vi "Core-GetTicks.vi"(8 "error in (no error)":errorcluster, 11 "Engine in":refnum<class "Engine.lvclass">) -> (0 "error out":errorcluster, 3 "Engine out":refnum<class "Engine.lvclass">)   [LabVIEW 2024, in "GLF.lvlib" / "Engine.lvclass"]
uses:
  Engine.lvclass
  Engine.lvclass/Engine.ctl
  <vilib>/Saukko/LV SDL3/Sources/SDL3/Timer/Timer.lvlib
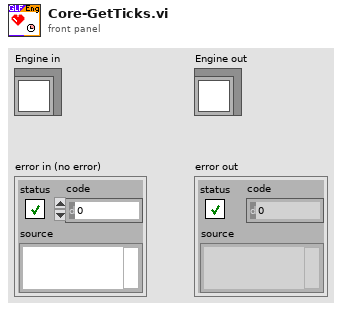
[diagram p1: front panel]
types:
  T1 = typedef "GLF.lvlib/Engine.lvclass/DVR--cluster.ctl" = cluster{"CMD Queue":T2, "Config":T3, "Ctxt":T5, "Metrics":T6, "GLF Instances":set{refnum<class "IAmGLF.lvclass">}, "Window Instances":map{i64, refnum<class "Window.lvclass">}}
  T2 = typedef "GLF.lvlib/Engine.lvclass/Command--queue.ctl" = refnum<queue>
  T3 = typedef "GLF.lvlib/Engine.lvclass/Config--cluster.ctl" = cluster{"Quit On Last Window Closed":bool, "VSync":T4, "FPS Target":dbl}
  T4 = typedef "GLF.lvlib/Engine.lvclass/VSync--enum.ctl" = enum16{"Disabled", "Enabled", "Adaptative"}
  T5 = typedef "GLF.lvlib/Engine.lvclass/Context--cluster.ctl" = cluster{"Ticks Begin":u64, "VSync Enabled":bool}
  T6 = typedef "GLF.lvlib/Engine.lvclass/Metrics--cluster.ctl" = cluster{"Uptime [ms]":u64, "Loop Time [ms]":u64}
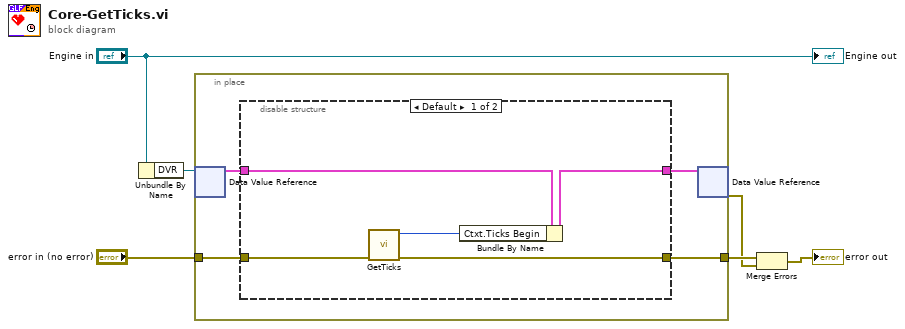
[diagram p0: block diagram]
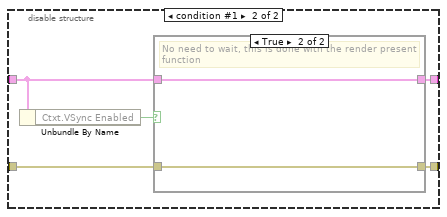
[diagram p2: hidden frame]
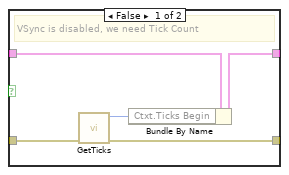
[diagram p3: hidden frame]
diagram:
  n1 = Unbundle By Name("Engine in") -> ("DVR"=w3:refnum<data-value>)
  n2 = in-place {
    in-place-border: "error in (no error)" -> [w10]
    in-place-border: [w9] -> w5
    n3 = in-place-dvr #1(w3) -> (w8:T1)  [unwired: 1 out]
    n4 = disable-structure shown="Default" {
      disable-tunnel: w10 -> [w15 w20]
      disable-tunnel: w8 -> [w12 w17]
      disable-tunnel: [w11 w19] -> w7
      disable-tunnel: [w13 w18] -> w9
      frame condition #0 (active) {
        n5 = call <vilib>:"GetTicks.vi"("No Error"=w15) -> ("error out"=w13:errorcluster, "Ticks [ms]"=w14:u64)  [unwired: 9 in]
        n6 = Bundle By Name(cluster=w12, "Ctxt.Ticks Begin"=w14) -> (w11:T1)
      }
      frame condition #1 {
        n7 = Unbundle By Name(w17) -> ("Ctxt.VSync Enabled"=w16:bool)
        n8 = case shown="True" w16 {
          tunnel: w20 -> [w25 w26]
          tunnel: w17 -> [w24 w27]
          tunnel: [w23 w27] -> w19
          tunnel: [w21 w26] -> w18
          frame False {
            # "VSync is disabled, we need Tick Count"
            n9 = call <vilib>:"GetTicks.vi"("No Error"=w25) -> ("error out"=w21:errorcluster, "Ticks [ms]"=w22:u64)  [unwired: 9 in]
            n10 = Bundle By Name(cluster=w24, "Ctxt.Ticks Begin"=w22) -> (w23:T1)
          }
          frame True {
            # "No need to wait, this is done with the render present function"
          }
        }
      }
    }
    n11 = in-place-dvr #1(w7) -> (w1:errorcluster)  [unwired: 1 out]
  }
  n12 = Merge Errors(w5, w1) -> (→"error out":errorcluster)
  "Engine out" <- "Engine in"
